vi "Unsubscribe.vi"(6 "Time out (ms)":i32=1000, 7 "Topic":string, 8 "error in (no error)":errorcluster, 9 "WAMP Client in":refnum<class "WAMP Client.lvclass">) -> (1 "Success?":bool, 2 "error out":errorcluster, 3 "WAMP Client out":refnum<class "WAMP Client.lvclass">)   [LabVIEW 2020, in "wamplv.lvlib" / "WAMP Client.lvclass"]
uses:
  <vilib>/samangh/wamplv/WAMP Client/WAMP Client.lvclass
  <vilib>/Utility/error.llb/Error Cluster From Error Code.vi
  <vilib>/ErrorRing/Error Ring.xnode
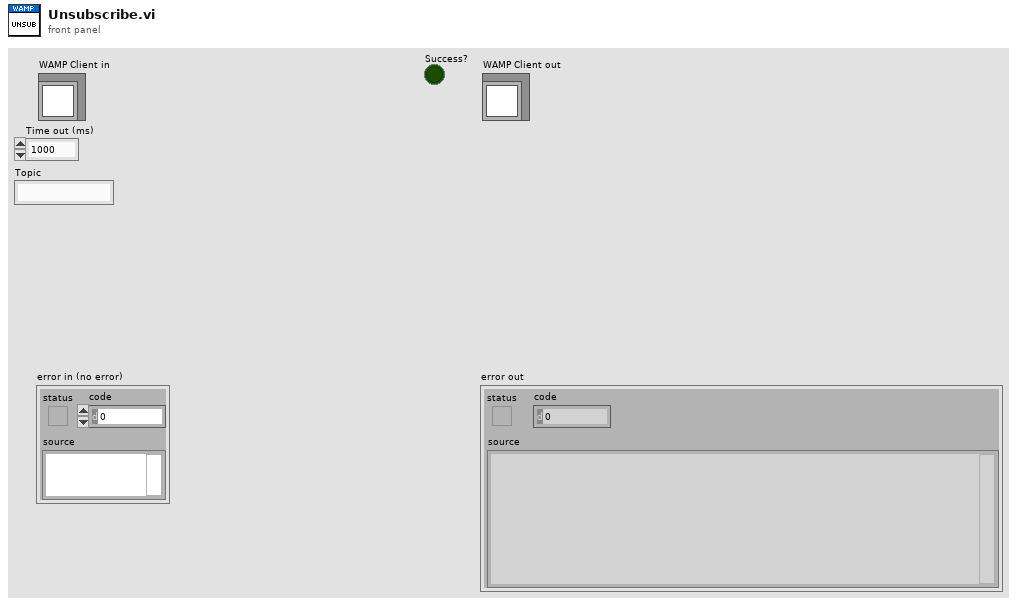
[diagram p1: front panel]
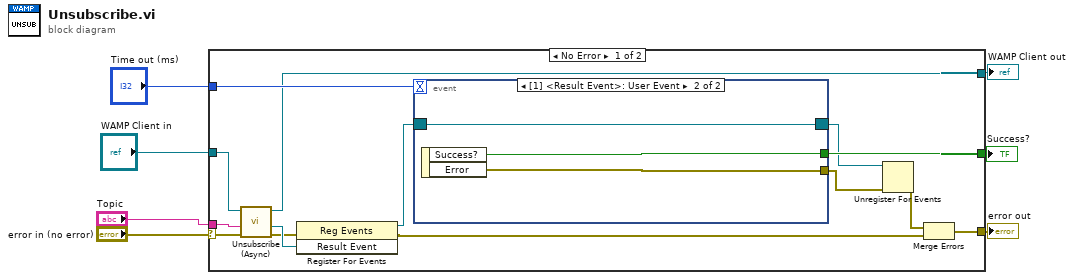
[diagram p0: block diagram]
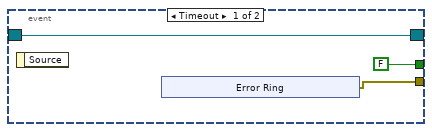
[diagram p2: hidden frame]
diagram:
  n1 = case shown="No Error" "error in (no error)" {
    selector: "error in (no error)" -> [w8 w34]
    tunnel: [w14 w34] -> w7
    tunnel: [w15 w33] -> w5
    tunnel: "WAMP Client in" -> [w18 w33]
    tunnel: [w20 _] -> w4
    tunnel: "Time out (ms)" -> [w19 _]
    tunnel: "Topic" -> [w17 _]
    frame No Error {
      n2 = call-dynamic "Unsubscribe (Async).vi"("error in (no error)"=w8, "Topic"=w17, "WAMP Client in"=w18) -> ("error out"=w9:errorcluster, "Result Event"=w16:refnum<user-event>, "WAMP Client out"=w15:refnum<class "WAMP Client.lvclass">)  [unwired: 6 in]
      n3 = register-events(error in=w9, w16) -> (reference out=w21:refnum<event-registration>, error out=w13:errorcluster)  [unwired: 1 in]
      n4 = event shown="[1] <Result Event>: User Event" {
        selector: w21 -> [w23 w30]
        dyn-events: [w23 w30] -> w10
        timeout: w19 -> [_ _]
        tunnel: [FALSE ("Success?") w32] -> w20
        tunnel: [w22 w31] -> w12
        event Timeout {
          n5 = event-data() -> ()  [unwired: 1 in, 1 out]
          n6 = xnode "Error Ring"() -> ("error out"=w22:errorcluster)
        }
        event User Event {
          n7 = event-data() -> ("Success?"=w32:bool, "Error"=w31:errorcluster)  [unwired: 1 in]
        }
      }
      n8 = Unregister For Events(event registration refnum=w10, error in=w12) -> (error out=w11:errorcluster)
      n9 = Merge Errors(w11, w13) -> (w14:errorcluster)
    }
    frame Error {
    }
  }
  "error out" <- w7
  "WAMP Client out" <- w5
  "Success?" <- w4
